vi "JL_Heat Data_Transfer.vi"(10 "Heat Control in":T2, 11 "Heat Control out 3":T1) -> (3 "Heat Control out":T1)   [LabVIEW 2016]
uses:
  Controls/Auto_Heat Control_Out.ctl
  Tools/Laundry/JL Dryer Tool/JL Dryer Tool Support/type defs/Heat Control.ctl
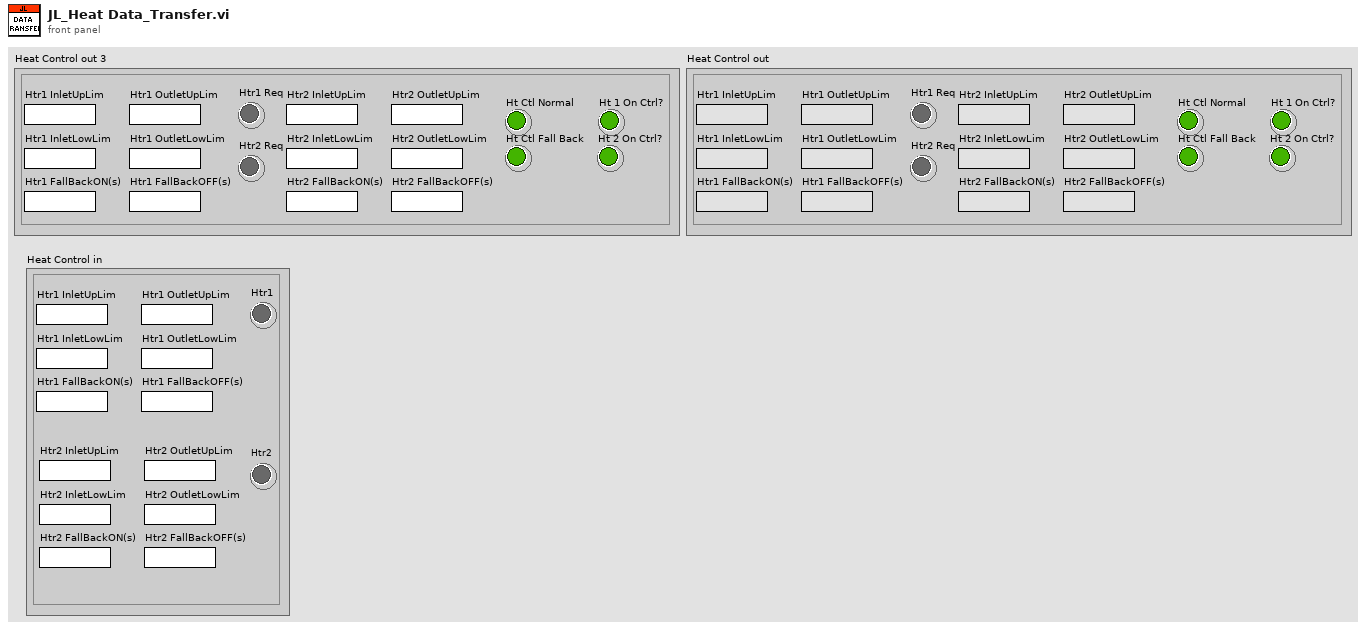
[diagram p1: front panel]
types:
  T1 = typedef "Auto_Heat Control_Out.ctl" = cluster{"Htr1 InletLowLim":string, "Htr1 InletUpLim":string, "Htr1 OutletLowLim":string, "Htr1 OutletUpLim":string, "Htr1 FallBackON(s)":string, "Htr1 FallBackOFF(s)":string, "Htr1 Req":bool, "Htr2 InletLowLim":string, "Htr2 InletUpLim":string, "Htr2 OutletLowLim":string, "Htr2 OutletUpLim":string, "Htr2 FallBackON(s)":string, "Htr2 FallBackOFF(s)":string, "Htr2 Req":bool, "Ht Ctl Normal":bool, "Ht Ctl Fall Back":bool, "Ht 1 On Ctrl?":bool, "Ht 2 On Ctrl?":bool}
  T2 = typedef "Heat Control.ctl" = cluster{"Htr1 InletLowLim":string, "Htr1 InletUpLim":string, "Htr1 OutletLowLim":string, "Htr1 OutletUpLim":string, "Htr1 FallBackON(s)":string, "Htr1 FallBackOFF(s)":string, "Htr1":bool, "Htr2 InletLowLim":string, "Htr2 InletUpLim":string, "Htr2 OutletLowLim":string, "Htr2 OutletUpLim":string, "Htr2 FallBackON(s)":string, "Htr2 FallBackOFF(s)":string, "Htr2":bool}
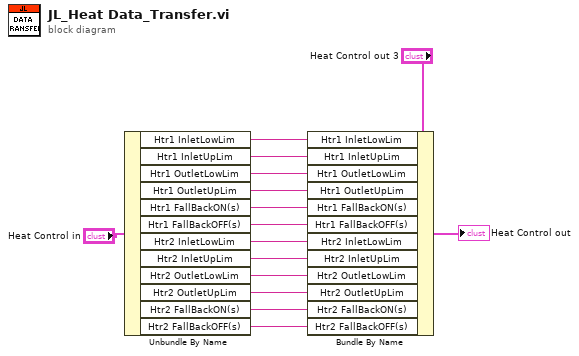
[diagram p0: block diagram]
diagram:
  n1 = Unbundle By Name("Heat Control in") -> ("Htr1 InletLowLim"=w14:string, "Htr1 InletUpLim"=w1:string, "Htr1 OutletLowLim"=w2:string, "Htr1 OutletUpLim"=w3:string, "Htr1 FallBackON(s)"=w4:string, "Htr1 FallBackOFF(s)"=w5:string, "Htr2 InletLowLim"=w6:string, "Htr2 InletUpLim"=w7:string, "Htr2 OutletLowLim"=w8:string, "Htr2 OutletUpLim"=w9:string, "Htr2 FallBackON(s)"=w10:string, "Htr2 FallBackOFF(s)"=w11:string)
  n2 = Bundle By Name(cluster="Heat Control out 3", "Htr1 InletLowLim"=w14, "Htr1 InletUpLim"=w1, "Htr1 OutletLowLim"=w2, "Htr1 OutletUpLim"=w3, "Htr1 FallBackON(s)"=w4, "Htr1 FallBackOFF(s)"=w5, "Htr2 InletLowLim"=w6, "Htr2 InletUpLim"=w7, "Htr2 OutletLowLim"=w8, "Htr2 OutletUpLim"=w9, "Htr2 FallBackON(s)"=w10, "Htr2 FallBackOFF(s)"=w11) -> (→"Heat Control out":T1)
